vi "fft_transfer.vi"(1 "Sample Rate":i32, 2 "Transfer Function":cdb[](array[numeric]), 3 "GRF Output":dbl[](array[numeric])) -> (0 "GRF Input":dbl[](array[numeric]))   [LabVIEW 2012]
uses:
  <vilib>/Analysis/2dsp.llb/Real FFT.vi
  <vilib>/Analysis/2dsp.llb/Inverse Real FFT.vi
  <vilib>/Analysis/3filter.llb/Butterworth Filter (DBL).vi
  <vilib>/Analysis/NI_AALPro.lvlib
  <vilib>/Analysis/NI_AALBase.lvlib
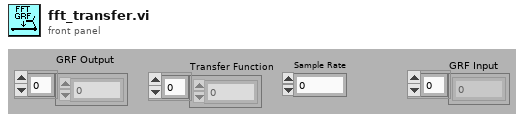
[diagram p1: front panel]
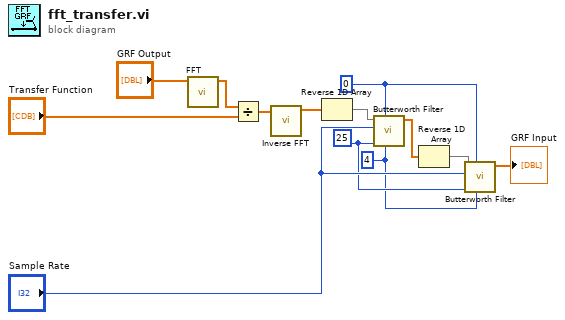
[diagram p0: block diagram]
diagram:
  w1 = 0
  w3 = 25
  w2 = 4
  n1 = call-poly <vilib>:"FFT.vi"("X"="GRF Output") -> ("FFT {X}"=w5:cdb[])  [unwired: 9 in, 1 out]
  n2 = Divide(x=w5, y="Transfer Function") -> (x/y=w7:cdb[])
  n3 = call-poly <vilib>:"Inverse FFT.vi"("FFT {X}"=w7) -> ("X"=w11:dbl[])  [unwired: 9 in, 1 out]
  n4 = Reverse 1D Array(array=w11) -> (reversed array=w8:dbl[])
  n5 = call-poly <vilib>:"Butterworth Filter.vi"("order"=w2, "filter type"=w1, "low cutoff freq: fl"=w3, "sampling freq: fs"="Sample Rate", "X"=w8) -> ("Filtered X"=w9:dbl[])  [unwired: 3 in, 1 out]
  n6 = Reverse 1D Array(array=w9) -> (reversed array=w10:dbl[])
  n7 = call-poly <vilib>:"Butterworth Filter.vi"("order"=w2, "filter type"=w1, "low cutoff freq: fl"=w3, "sampling freq: fs"="Sample Rate", "X"=w10) -> ("Filtered X"=→"GRF Input":dbl[])  [unwired: 3 in, 1 out]
